vi "sv_Test Weighting Filter.vi"(6 "type or class":enum16{"Type 0 / Class 1", "Type 1 / Class 2"}(ring)=enum."Type 1 / Class 2", 7 "standard":enum16{"ANSI S1.4", "IEC 61672"}(ring), 8 "error in (no error)":errorcluster, 9 "filter coefficients":T1 {"Forward Coefficients" format="%.4f"; "Reverse Coefficients" format="%.4f"}, 10 "weighting":u16(ring) items=["Linear", "A-weighting", "B-weighting", "C-weighting"], 11 "sampling frequency [Hz]":dbl=10000.0 format="%.2f") -> (0 "error out":errorcluster, 3 "max freq within tolerances [Hz]":dbl format="%.2f")   [LabVIEW 2017]
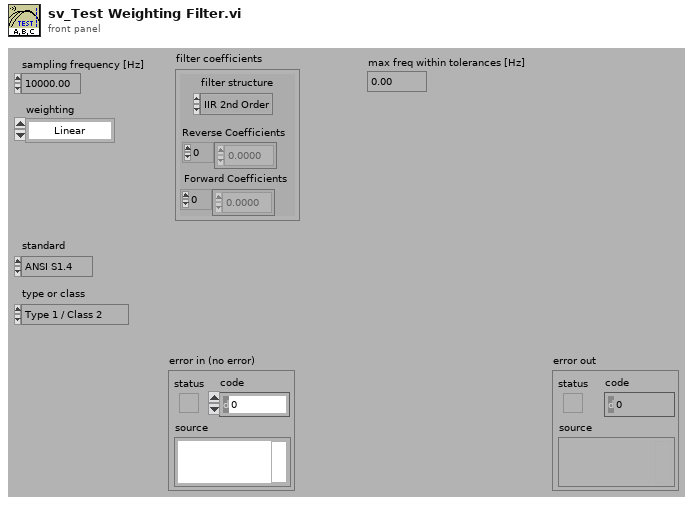
[diagram p1: front panel]
types:
  T1 = cluster{"filter structure":enum32{"IIR 2nd Order", "IIR 4th Order"}, "Reverse Coefficients":dbl[], "Forward Coefficients":dbl[]}
  T2 = typedef "svc_Weighting Filter Text Ring.ctl" = u16
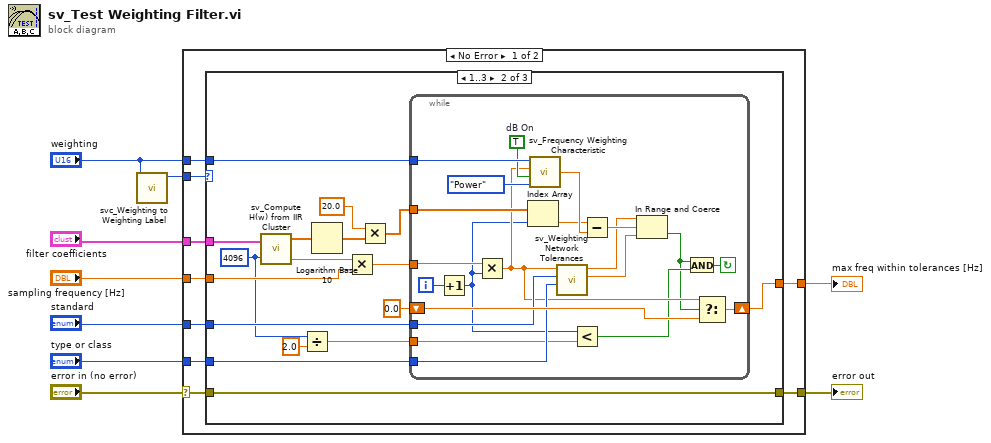
[diagram p0: block diagram]
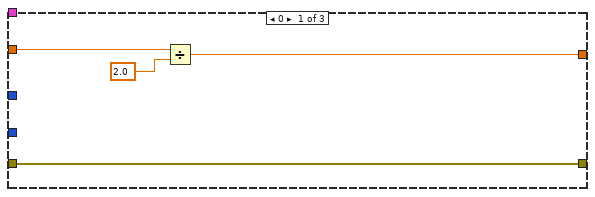
[diagram p2: hidden frame]
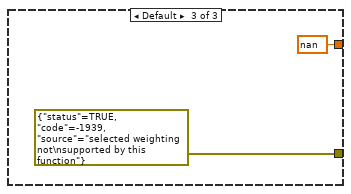
[diagram p3: hidden frame]
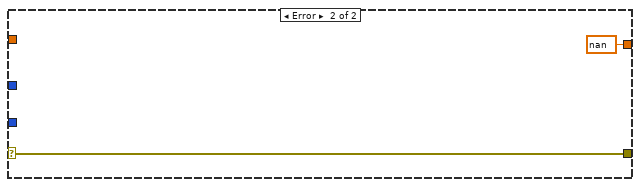
[diagram p4: hidden frame]
diagram:
  n1 = call <vilib>:"svc_Weighting to Weighting Label.vi"("weighting filter"="weighting") -> ("weighting enum"=w1:T2)  [unwired: 9 in, 1 out]
  n2 = case shown="No Error" "error in (no error)" {
    selector: "error in (no error)" -> [w10 w64]
    tunnel: "sampling frequency [Hz]" -> [w18 _]
    tunnel: "weighting" -> [w13 _]
    tunnel: [w17 nan] -> w8
    tunnel: [w11 w64] -> w6
    tunnel: "filter coefficients" -> [w16 _]
    tunnel: "standard" -> [w15 _]
    tunnel: "type or class" -> [w14 _]
    tunnel: w1 -> [w12 _]
    frame No Error {
      n3 = case shown="1..3" w12 {
        tunnel: w18 -> [w22 w35 _]
        tunnel: [w20 w32 nan] -> w17
        tunnel: w16 -> [_ w31 _]
        tunnel: w15 -> [_ w30 _]
        tunnel: w14 -> [_ w29 _]
        tunnel: w13 -> [_ w27 _]
        tunnel: [w19 w23 errorcluster {"status"=TRUE, "code"=-1939, "source"="selected weighting not\nsupported by this function"} ("error out")] -> w11
        tunnel: w10 -> [w19 w23 _]
        frame 0 {
          n4 = Divide(x=w22, y=2.0) -> (x/y=w20:dbl)
        }
        frame 1..3 {
          w26 = 4096 ("FFT size")
          n5 = call <vilib>:"sv_Compute H(w) from IIR Cluster.vi"("filter coefficients"=w31, "FFT size"=w26) -> ("mag H(w)"=w36:dbl[], "df"=w39:dbl)  [unwired: 1 out]
          n6 = Divide(x=w26, y=2.0) -> (x/y=w24:dbl)
          n7 = Logarithm Base 10(1:w36) -> (0:w37:dbl[])
          n8 = Multiply(x=w39, y=w35) -> (x*y=w34:dbl)
          n9 = Multiply(x=20.0, y=w37) -> (x*y=w33:dbl[])
          n10 = while {
            tunnel: w30 -> [w49]
            shift-left: 0.0 -> [w54]
            shift-right: [w53] -> w32
            tunnel: w33 -> [w52]
            tunnel: w34 -> [w59]
            tunnel: w27 -> [w60]
            tunnel: w29 -> [w48]
            tunnel: w24 -> [w42]
            i -> [w50]
            stop <- w44 continue-if-true
            w58 = TRUE  # dB On
            n11 = Increment(x=w50) -> (x+1=w43:i32)
            n12 = Multiply(x=w59, y=w43) -> (x*y=w45:dbl)
            n13 = Index Array(array=w52, index=w43) -> (element=w51:dbl)
            n14 = call <vilib>:"sv_Frequency Weighting Characteristic.vi"("spectrum type"=enum16{"Power", "Amplitude"}."Power", "dB On (T)"=w58, "frequency [Hz]"=w45, "weighting filter"=w60) -> ("relative response level"=w56:dbl)
            n15 = call <vilib>:"sv_Weighting Network Tolerances.vi"("type or class"=w48, "standard"=w49, "frequency [Hz]"=w45) -> ("low tolerance [dB]"=w46:dbl, "high tolerance [dB]"=w47:dbl)  [unwired: 7 in]
            n16 = Less?(x=w43, y=w42) -> (x < y?=w41:bool)
            n17 = Subtract(x=w51, y=w56) -> (x-y=w55:dbl)
            n18 = In Range and Coerce(upper limit=w47, x=w55, lower limit=w46) -> (In Range?=w40:bool)  [unwired: 1 out]
            n19 = And(x=w40, y=w41) -> (x .and. y?=w44:bool)
            n20 = Select(t=w45, s=w40, f=w54) -> (s? t:f=w53:dbl)
          }
        }
        frame Default {
        }
      }
    }
    frame Error {
    }
  }
  "max freq within tolerances [Hz]" <- w8
  "error out" <- w6
